vi "Get Foreign Key.vi"(8 "error in (no error)":errorcluster, 9 "Column Name Array":string[](array[string]), 10 "Table Name":string, 11 "ADODB in":refnum<class "ADODB.lvclass">) -> (0 "error out":errorcluster, 2 "FK Properties Array":T1[](array[typedef]), 3 "ADODB out":refnum<class "ADODB.lvclass">)   [LabVIEW 2020, in "ADODB.lvclass"]
uses:
  ADODB.lvclass
  foreign key properties.ctl
  ADODB.lvclass/ADODB.ctl
  <vilib>/addons/database/NI_Database_API.lvlib
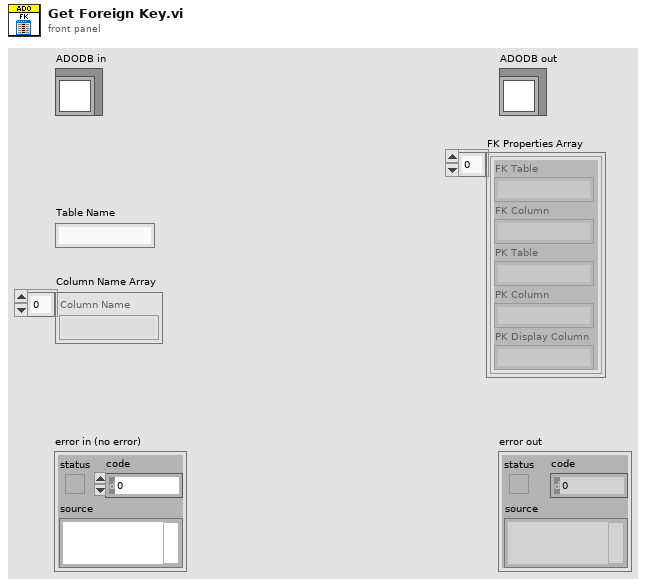
[diagram p1: front panel]
types:
  T1 = typedef "foreign key properties.ctl" = cluster{"FK Table":string, "FK Column":string, "PK Table":string, "PK Column":string, "PK Display Column":string}
  T2 = cluster{"Parent Table":string, "Parent Column":string, "Foreign Table":string, "Foreign PK Column":string, "Foreign Display Column":string}[]
  T3 = typedef "NI_Database_API.lvlib/Conn ObjectReference.ctl" = refnum<k1>
  T4 = typedef "NI_Database_API.lvlib/Conn DataMembers.ctl" = cluster{"ADODB._Connection":refnum<k7>, "recordset objects":i32, "command objects":i32}
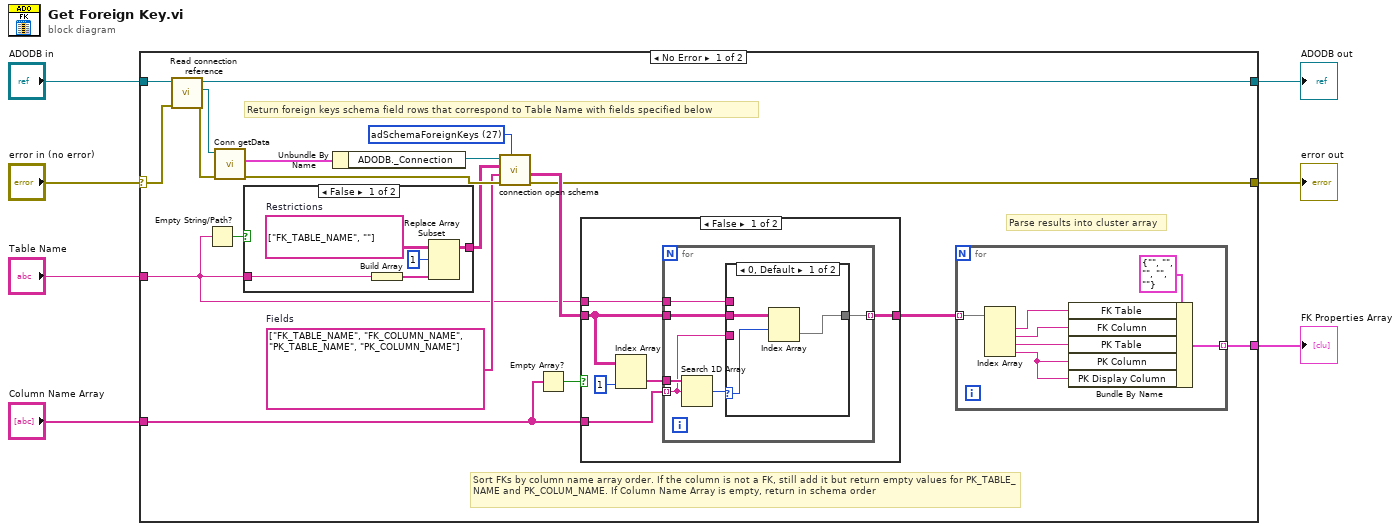
[diagram p0: block diagram]
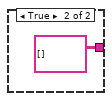
[diagram p2: hidden frame]
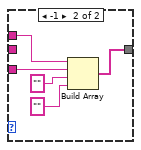
[diagram p3: hidden frame]
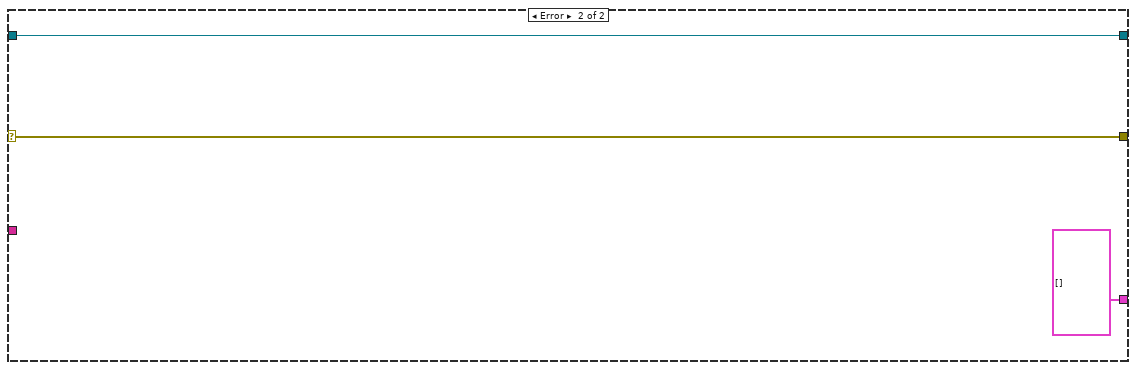
[diagram p5: hidden frame]
diagram:
  n1 = case shown="No Error" "error in (no error)" {
    selector: "error in (no error)" -> [w20 w63]
    tunnel: "ADODB in" -> [w22 w62]
    tunnel: [w21 w62] -> w6
    tunnel: [w19 T2 []] -> w1
    tunnel: "Table Name" -> [w9 _]
    tunnel: "Column Name Array" -> [w13 _]
    tunnel: [w10 w63] -> w2
    frame No Error {
      w16 = string[] ["FK_TABLE_NAME", "FK_COLUMN_NAME", "PK_TABLE_NAME", "PK_COLUMN_NAME"]  # Fields
      w17 = 27 items=["adSchemaProviderSpecific"=-1, "adSchemaAsserts"=0, "adSchemaCatalogs"=1, "adSchemaCharacterSets"=2, "adSchemaCollations"=3, "adSchemaColumns"=4, "adSchemaCheckConstraints"=5, "adSchemaConstraintColumnUsage"=6, "adSchemaConstraintTableUsage"=7, "adSchemaKeyColumnUsage"=8, "adSchemaReferentialContraints, adSchemaReferentialConstraints"=9, "adSchemaTableConstraints"=10, "adSchemaColumnsDomainUsage"=11, "adSchemaIndexes"=12, "adSchemaColumnPrivileges"=13, "adSchemaTablePrivileges"=14, "adSchemaUsagePrivileges"=15, "adSchemaProcedures"=16, "adSchemaSchemata"=17, "adSchemaSQLLanguages"=18, "adSchemaStatistics"=19, "adSchemaTables"=20, "adSchemaTranslations"=21, "adSchemaProviderTypes"=22, "adSchemaViews"=23, "adSchemaViewColumnUsage"=24, "adSchemaViewTableUsage"=25, "adSchemaProcedureParameters"=26, "adSchemaForeignKeys"=27, "adSchemaPrimaryKeys"=28, "adSchemaProcedureColumns"=29, "adSchemaDBInfoKeywords"=30, "adSchemaDBInfoLiterals"=31, "adSchemaCubes"=32, "adSchemaDimensions"=33, "adSchemaHierarchies"=34, "adSchemaLevels"=35, "adSchemaMeasures"=36, "adSchemaProperties"=37, "adSchemaMembers"=38, "adSchemaTrustees"=39] ("Schema")
      # "Return foreign keys schema field rows that correspond to Table Name with fields specified below"
      # "Sort FKs by column name array order. If the column is not a FK, still add it but return empty values for PK_TABLE_NAME and PK_COLUM_NAME. If Column Name Array is empty, return in schema order"
      # "Parse results into cluster array"
      n2 = call "Read connection reference.vi"("error in (no error)"=w20, "ODBC in"=w22) -> ("error out"=w24:errorcluster, "reference"=w23:T3, "ODBC out"=w21:refnum<class "ADODB.lvclass">)  [unwired: 7 in]
      n3 = Empty String/Path?(string/path=w9) -> (empty?=w8:bool)
      n4 = call <vilib>:"Conn getData.vi"("error in (no error)"=w24, "connection reference"=w23) -> ("error out"=w18:errorcluster, "data"=w25:T4)  [unwired: 2 in, 2 out]
      n5 = case shown="False" w8 {
        tunnel: [w28 string[][] [] ("Restrictions")] -> w15
        tunnel: w9 -> [w27 _]
        frame False {
          w31 = string[][] [["FK_TABLE_NAME"], [""]]  # Restrictions
          n6 = Build Array(w27) -> (w29:string[])
          n7 = Replace Array Subset(array=w31, new element=w29, index (row)=1) -> (w28:string[][])  [unwired: 1 in]
        }
        frame True {
        }
      }
      n8 = Unbundle By Name(w25) -> ("ADODB._Connection"=w26:refnum<k7>)
      n9 = call "connection open schema.vi"("Schema"=w17, "error in (no error)"=w18, "Fields"=w16, "Restrictions"=w15, "ADODB._Connection"=w26) -> ("error out"=w10:errorcluster, "Schema Out"=w12:string[][])  [unwired: 3 in, 2 out]
      n10 = Empty Array?(array=w13) -> (empty?=w14:bool)
      n11 = case shown="False" w14 {
        tunnel: w12 -> [w37 w53]
        tunnel: w13 -> [w38 _]
        tunnel: [w33 w53] -> w11
        tunnel: w9 -> [w34 _]
        frame False {
          n12 = Index Array(array=w37, index (col)=1 ("disabled index (col)")) -> (element=w36:string[])  [unwired: 1 in]
          n13 = for {
            tunnel: w38 -> [w40] mode=indexing
            tunnel: w37 -> [w42]
            tunnel: w36 -> [w44]
            tunnel: w34 -> [w41]
            tunnel: [w39] -> w33 mode=indexing
            n14 = Search 1D Array(1D array=w44, element=w40) -> (index of element=w43:i32)  [unwired: 1 in]
            n15 = case shown="0, Default" w43 {
              selector: w43 -> [w46 _]
              tunnel: w42 -> [w47 _]
              tunnel: w41 -> [_ w52]
              tunnel: w40 -> [_ w49]
              tunnel: [w45 w48] -> w39
              frame 0, Default {
                n16 = Index Array(array=w47, index (row)=w46) -> (element=w45:string[])  [unwired: 1 in]
              }
              frame -1 {
                n17 = Build Array(w52, w49, "" ("element"), "" ("element")) -> (w48:string[])
              }
            }
          }
        }
        frame True {
        }
      }
      n18 = for {
        tunnel: [w60] -> w19 mode=indexing
        tunnel: w11 -> [w59] mode=indexing
        n19 = Index Array(array=w59) -> (element #1=w58:string, element #2=w57:string, element #3=w56:string, element #4=w55:string)  [unwired: 4 in]
        n20 = Bundle By Name(cluster=T1 {"FK Table"="", "FK Column"="", "PK Table"="", "PK Column"="", "PK Display Column"=""} ("Foreign Key"), "FK Table"=w58, "FK Column"=w57, "PK Table"=w56, "PK Column"=w55, "PK Display Column"=w55) -> (w60:T1)
      }
    }
    frame Error {
    }
  }
  "error out" <- w2
  "ADODB out" <- w6
  "FK Properties Array" <- w1
